vi "flow_queue_init.vi"(8 "error in (no error)":errorcluster caption="エラー入力（エラーなし）", 11 "queue config":T1(array[cluster])) -> (0 "error out":errorcluster caption="エラー出力", 3 "flow_refnum":refnum<queue>[](array[refnum]))   [LabVIEW 2017]
uses:
  flow_queue_datatype.ctl
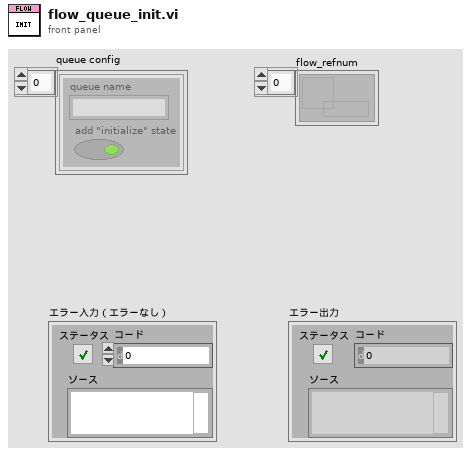
[diagram p1: front panel]
types:
  T1 = cluster{"queue name":string, "add \"initialize\" state":bool}[]
  T2 = typedef "flow_queue_datatype.ctl" = cluster{"command":string, "parameter":variant}
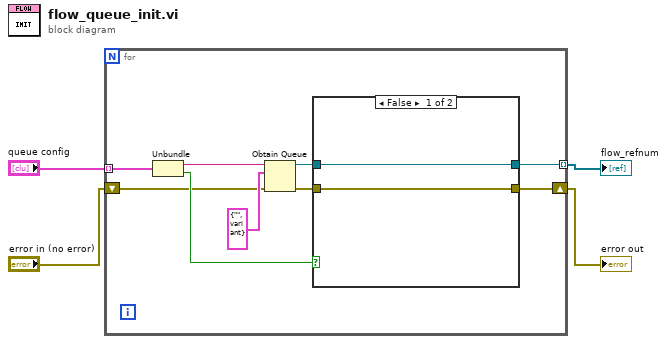
[diagram p0: block diagram]
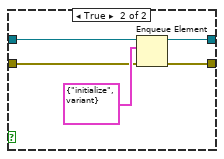
[diagram p2: hidden frame]
diagram:
  n1 = for {
    tunnel: "queue config" -> [w13] mode=indexing
    shift-right: [w6] -> w2
    shift-left: "error in (no error)" -> [w7]
    tunnel: [w5] -> w1 mode=indexing
    n2 = Unbundle(w13) -> ("queue name"=w12:string, "add \"initialize\" state"=w10:bool)
    n3 = Obtain Queue(name (unnamed)=w12, element data type=T2 {"command"="", "parameter"=variant} ("flow_control_3_datatype"), error in (no error)=w7) -> (queue out=w11:refnum<queue>, error out=w9:errorcluster)  [unwired: 2 in, 1 out]
    n4 = case shown="False" w10 {
      tunnel: w11 -> [w14 w20]
      tunnel: w9 -> [w15 w18]
      tunnel: [w15 w17] -> w6
      tunnel: [w14 w16] -> w5
      frame False {
      }
      frame True {
        n5 = Enqueue Element(queue=w20, element=T2 {"command"="initialize", "parameter"=variant} ("flow_control_3_datatype"), error in (no error)=w18) -> (queue out=w16:refnum<queue>, error out=w17:errorcluster)  [unwired: 1 in, 1 out]
      }
    }
  }
  "error out" <- w2
  "flow_refnum" <- w1
